vi "Test Process Trigger Broadcast.vi"(8 "error in (no error)":errorcluster, 11 "Process Test In":refnum<class "Process Test.lvclass">) -> (0 "error out":errorcluster, 3 "Process Test Out":refnum<class "Process Test.lvclass">)   [LabVIEW 2020, in "Process Test.lvclass"]
uses:
  Process Test.lvclass
  Framework/Process/Process.lvclass
  Support/Event Helpers/Event Helpers.lvlib
  <vilib>/Asteme/LUnit/Test Case.lvclass
  C:/Users/anton/Documents/GitHub/Triarc-Framework/source/Framework Test/Base Class Test/Base Test.lvclass
  C:/Program Files (x86)/National Instruments/LabVIEW 2020/vi.lib/Asteme/LUnit/Test Case.lvclass
  C:/Users/anton/Documents/GitHub/Triarc-Framework/source/Framework Test/Process Test/Process Test.lvclass
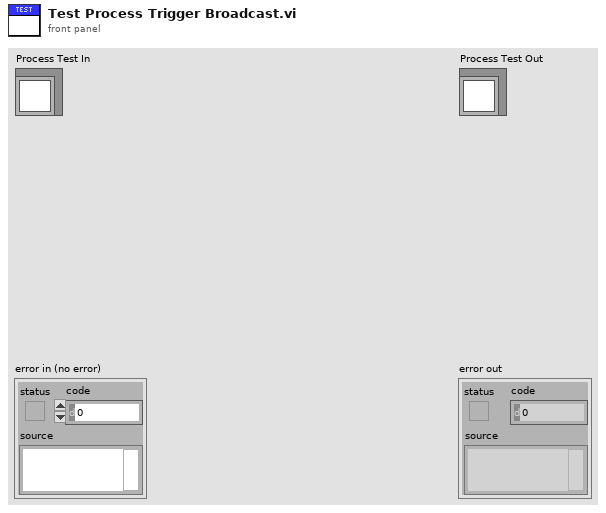
[diagram p1: front panel]
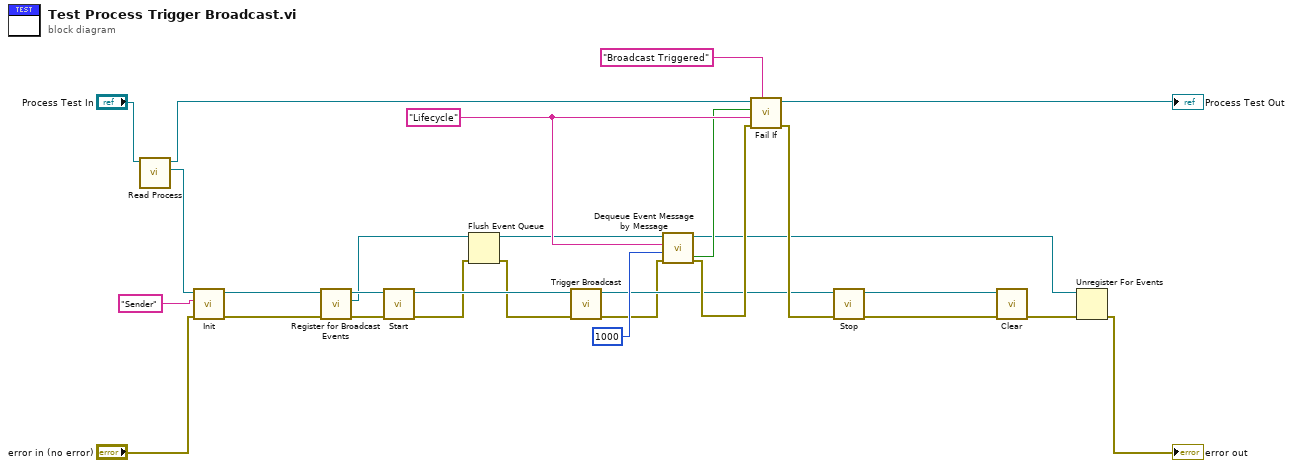
[diagram p0: block diagram]
diagram:
  w12 = "Lifecycle" ("Message")
  n1 = call "Read Process.vi"("Process Test in"="Process Test In") -> ("Process.lvclass"=w21:refnum<class "Process.lvclass">, "Process Test out"=w7:refnum<class "Process Test.lvclass">)  [unwired: 8 in, 1 out]
  n2 = call-dynamic "Init.vi"("error in (no error)"="error in (no error)", "Name"="Sender" ("Message"), "Process In"=w21) -> ("error out"=w27:errorcluster, "Process Out"=w28:refnum<class "Process.lvclass">)  [unwired: 7 in]
  n3 = call-dynamic "Register for Broadcast Events.vi"("error in (no error)"=w27, "Process In"=w28) -> ("error out"=w19:errorcluster, "Event Registration Refnum"=w6:refnum<event-registration>, "Process Out"=w20:refnum<class "Process.lvclass">)  [unwired: 7 in]
  n4 = call "Start.vi"("error in (no error)"=w19, "Process In"=w20) -> ("error out"=w4:errorcluster, "Process Out"=w18:refnum<class "Process.lvclass">)  [unwired: 8 in]
  n5 = Flush Event Queue(0:w6, 3:w4) -> (8:w5:refnum<event-registration>, 11:w2:errorcluster)  [unwired: 4 in, 1 out]
  n6 = call "Trigger Broadcast.vi"("error in (no error)"=w2, "Process in"=w18) -> ("error out"=w1:errorcluster, "Process out"=w3:refnum<class "Process.lvclass">)  [unwired: 8 in]
  n7 = call "Dequeue Event Message by Message.vi"("error in (no error)"=w1, "Timeout (-1)"=1000, "Message"=w12, "Event Registration Refnum"=w5) -> ("error out"=w13:errorcluster, "Event Registration Refnum Out"=w9:refnum<event-registration>, "Timed Out?"=w11:bool)  [unwired: 3 in, 2 out]
  n8 = call <vilib>:"Fail If.vi"("Description"="Broadcast Triggered", "error in (no error)"=w13, "Message"=w12, "Fail?"=w11, "Test Case In"=w7) -> ("error out"=w14:errorcluster, "Test Case Out"=→"Process Test Out":refnum<class "Process Test.lvclass">)  [unwired: 5 in]
  n9 = call "Stop.vi"("error in (no error)"=w14, "Process In"=w3) -> ("error out"=w16:errorcluster, "Process Out"=w26:refnum<class "Process.lvclass">)  [unwired: 7 in, 1 out]
  n10 = call-dynamic "Clear.vi"("error in (no error)"=w16, "Process In"=w26) -> ("error out"=w25:errorcluster)  [unwired: 8 in, 1 out]
  n11 = Unregister For Events(event registration refnum=w9, error in=w25) -> (error out=→"error out":errorcluster)
